vi "Get Default Row.vi"(0 "ItemNames":string[][](array[string]), 7 "Columns":T1[](array[typedef])) -> (4 "Default Row":string[](array[string]), 8 "rings":i32[](array[numeric]), 10 "# rows":i32)   [LabVIEW 2020, in "KTable.xctl"]
uses:
  KTable.xctl
  ColumnSpec.ctl
  ColumnType.ctl
  Array Manipulation VIs/Array-Dimensions (2D string).vi
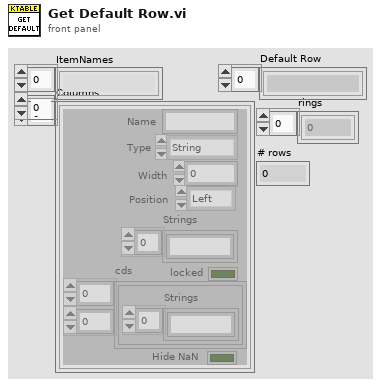
[diagram p1: front panel]
types:
  T1 = typedef "KTable.xctl/ColumnSpec.ctl" = cluster{"Name":string, "Type":T2, "Width":i32, "Strings":string[], "Position":enum16{"Left", "Center", "Right"}, "locked":bool, "cds":cluster{"Strings":string[]}[][], "Hide NaN":bool}
  T2 = typedef "KTable.xctl/ColumnType.ctl" = enum16{"String", "Enum", "Int", "Double", "Boolean", "Ring", "Formula", "Color"}
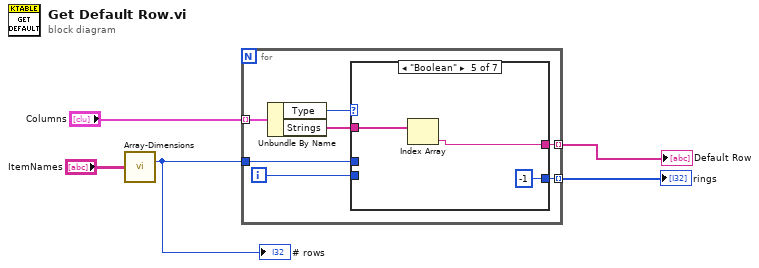
[diagram p0: block diagram]
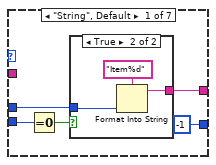
[diagram p2: hidden frame]
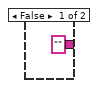
[diagram p3: hidden frame]
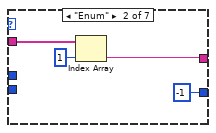
[diagram p4: hidden frame]
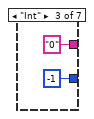
[diagram p5: hidden frame]
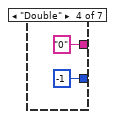
[diagram p6: hidden frame]
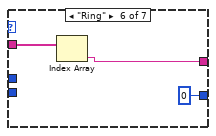
[diagram p7: hidden frame]
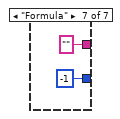
[diagram p8: hidden frame]
diagram:
  n1 = call-poly "Array-Dimensions.vi"("2D Array"="ItemNames") -> ("# rows"=w3:i32)  [unwired: 13 in, 1 out]
  "# rows" <- w3
  n2 = for {
    tunnel: "Columns" -> [w12] mode=indexing
    tunnel: w3 -> [w8]
    tunnel: [w7] -> w5 mode=indexing
    tunnel: [w6] -> w1 mode=indexing
    i -> [w9]
    n3 = Unbundle By Name(w12) -> ("Type"=w11:T2, "Strings"=w10:string[])
    n4 = case shown="\"Boolean\"" w11 {
      tunnel: w10 -> [_ w25 _ _ w32 w35 _]
      tunnel: w9 -> [w17 _ _ _ _ _ _]
      tunnel: w8 -> [w15 _ _ _ _ _ _]
      tunnel: [w14 w23 "0" ("String") "0" ("String") w31 w34 "" ("String")] -> w7
      tunnel: [-1 -1 -1 -1 -1 0 -1] -> w6
      frame "String", Default {
        n5 = Equal To 0?(x=w17) -> (x = 0?=w16:bool)
        n6 = case shown="True" w16 {
          tunnel: w15 -> [_ w21]
          tunnel: ["" w19] -> w14
          frame False {
          }
          frame True {
            n7 = Format Into String(format string="Item%d", w21) -> (resulting string=w19:string)  [unwired: 2 in, 1 out]
          }
        }
      }
      frame "Enum" {
        n8 = Index Array(array=w25, index=1) -> (element=w23:string)
      }
      frame "Int" {
      }
      frame "Double" {
      }
      frame "Boolean" {
        n9 = Index Array(array=w32) -> (element=w31:string)  [unwired: 1 in]
      }
      frame "Ring" {
        n10 = Index Array(array=w35) -> (element=w34:string)  [unwired: 1 in]
      }
      frame "Formula" {
      }
    }
  }
  "Default Row" <- w5
  "rings" <- w1
